vi "RenderPresent.vi"(8 "No Error":errorcluster, 11 "Renderer [SDL_Renderer *]":i64 format="%.0x") -> (0 "error out":errorcluster)   [LabVIEW 2026, in "SDL3.lvlib" / "Render.lvlib"]
doc: "<B>Summary</B>\nUpdate the screen with any rendering performed since the previous call.\n\n<B>Remarks</B>\nSDL's rendering functions operate on a backbuffer; that is, calling a rendering function such as <B>SDL_RenderLine()</B> does not directly put a line on the screen, but rather updates the backbuffer. As such, you compose your entire scene and present the composed backbuffer to the screen as a complete picture.\n\nTherefore, when using SDL's rendering API, one does all drawing intended for the frame, and then calls this function once per frame to present the final drawing to the user.\n\nThe backbuffer should be considered invalidated after each present; do not assume that previous contents will exist between frames. You are strongly encouraged to call <B>SDL_RenderClear()</B> to initialize the backbuffer before starting each new frame's drawing, even if you plan to overwrite every pixel.\n\nPlease note, that in case of rendering to a texture - there is no need to call SDL_RenderPresent after drawing needed objects to a texture, and should not be done; you are only required to change back the rendering target to default via <B>SDL_SetRenderTarget(renderer, NULL)</B> afterwards, as textures by themselves do not have a concept of backbuffers. Calling SDL_RenderPresent while rendering to a texture will still update the screen with any current drawing that has been done to the window itself."
uses:
  Render.lvlib
  <vilib>/Utility/error.llb/Error Cluster From Error Code.vi
  Error/Error.lvlib
  Lib/SDL3.dll
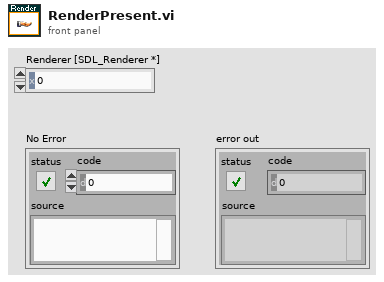
[diagram p1: front panel]
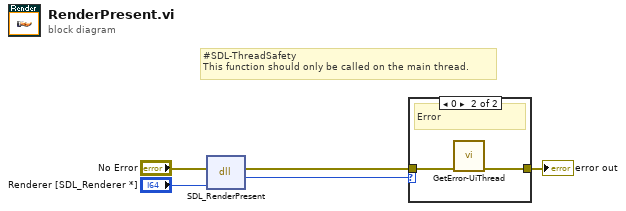
[diagram p0: block diagram]
diagram:
  # "#SDL-ThreadSafety\nThis function should only be called on the main thread."
  n1 = dll-call lib="C:/Users/saukko/Dev/LV-SDL3/Sources/SDL3/Lib/SDL3.*" fn="SDL_RenderPresent"(error in="No Error", "renderer"="Renderer [SDL_Renderer *]") -> (error out=w2:errorcluster, "return type"=w1:i32)  [unwired: 3 in, 1 out]
  n2 = case shown="0" w1 {
    tunnel: w2 -> [w6 w8]
    tunnel: [w6 w7] -> w4
    frame Default {
      # "Ok"
    }
    frame 0 {
      # "Error"
      n3 = call "GetError-UiThread.vi"("No Error"=w8) -> ("error out"=w7:errorcluster)  [unwired: 10 in]
    }
  }
  "error out" <- w4
